vi "TA_Status_Synchronous.vi"() -> ()   [LabVIEW 2025]
panel:
  out "data":dynamicdata(graph) caption="Status"
  in  "number of samples":i32=5000
  in  "rate":dbl=500000.0
  in  "stop (F)":bool
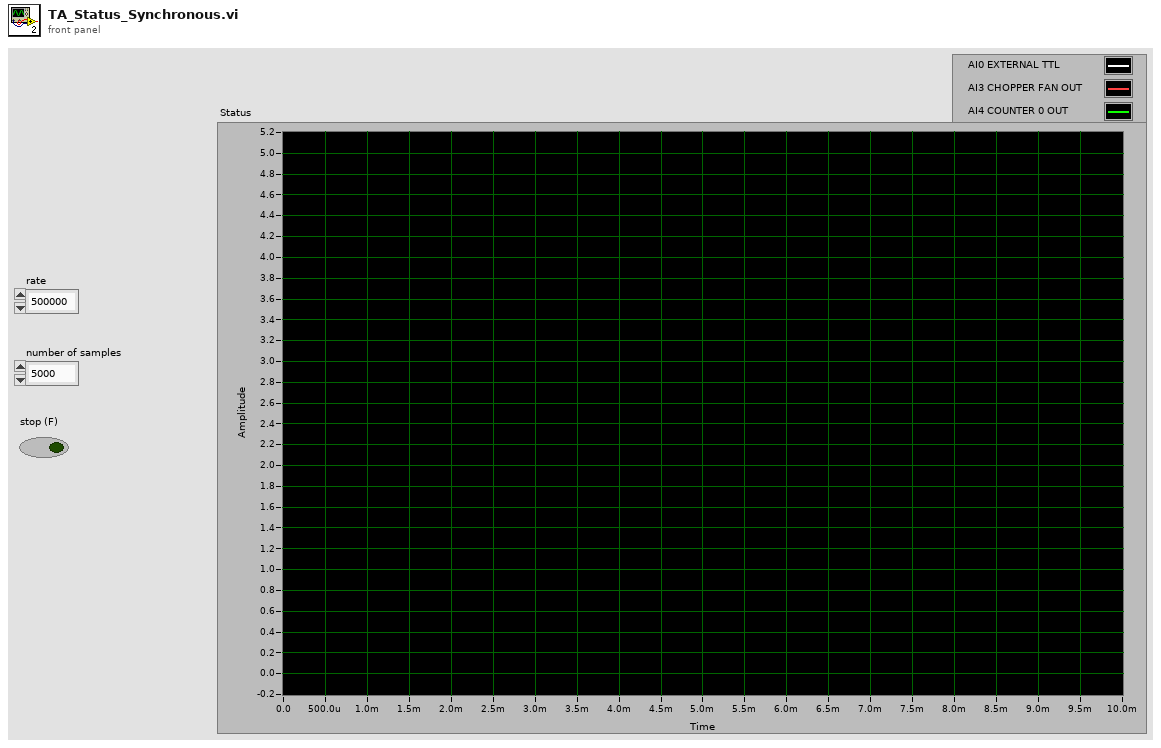
[diagram p1: front panel]
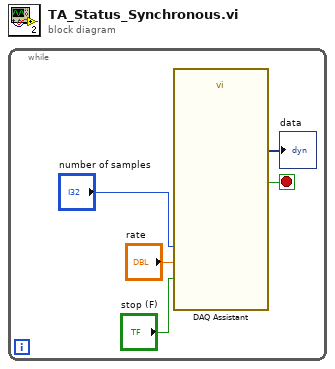
[diagram p0: block diagram]
diagram:
  n1 = while {
    stop <- w4 stop-if-true
    n2 = call "DAQ Assistant"("rate"="rate", "number of samples"="number of samples", "stop (F)"="stop (F)") -> ("data"=→"data":dynamicdata, "stopped"=w4:bool)  [unwired: 13 in, 2 out]
  }
